vi "UI_Progress.vi"(8 "error in (no error)":errorcluster, 11 "Progress in":refnum<class "Progress.lvclass">) -> (0 "error out":errorcluster, 3 "Progress out":refnum<class "Progress.lvclass">)   [LabVIEW 2021, in "Progress.lvlib" / "Progress.lvclass"]
uses:
  Progress.lvclass
panel:
  out "Slide":u64(slide) scale=0.0..1.0
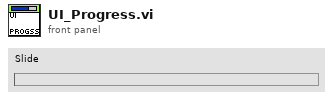
[diagram p1: front panel]
types:
  T1 = enum32{"Invalid", "Standard", "Closed", "Hidden", "Minimized", "Maximized"}
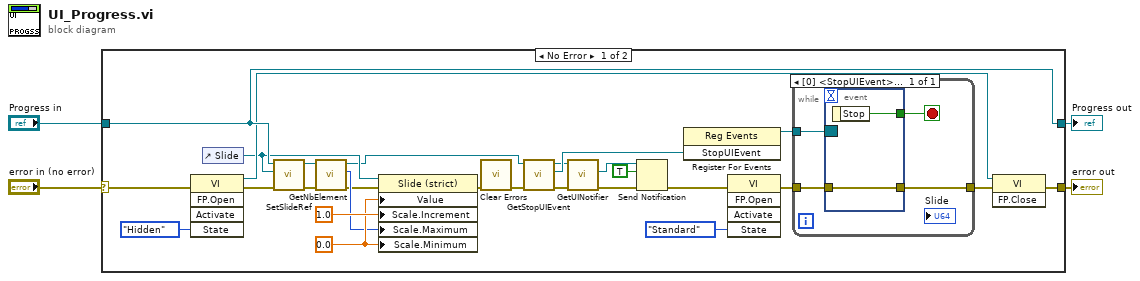
[diagram p0: block diagram]
diagram:
  n1 = case shown="No Error" "error in (no error)" {
    selector: "error in (no error)" -> [w16 w39]
    tunnel: [w15 w39] -> w3
    tunnel: [w31 w38] -> w1
    tunnel: "Progress in" -> [w31 w38]
    frame No Error {
      w13 = 0.0 ("ProgressValue")
      n2 = invoke class="VI" method="FP.Open"(error in=w16, "State"=T1."Hidden") -> (reference out=w18:refnum<vi>, error out=w19:errorcluster)  [unwired: 3 in, 3 out]
      n3 = control-ref of="Slide"() -> (w12:refnum<vi>)
      n4 = call "SetSlideRef.vi"("error in (no error)"=w19, "SlideRefnum"=w12, "Progress in"=w31) -> ("error out"=w11:errorcluster, "Progress out"=w10:refnum<class "Progress.lvclass">)  [unwired: 7 in]
      n5 = call "GetNbElement.vi"("error in (no error)"=w11, "Progress in"=w10) -> ("error out"=w6:errorcluster, "NbElement"=w9:u64, "Progress out"=w7:refnum<class "Progress.lvclass">)  [unwired: 7 in]
      n6 = property class="Slide (strict)"(reference=w12, error in=w6, "Value"=w13, "Scale.Increment"=1.0 ("Scale.Range:Increment"), "Scale.Maximum"=w9, "Scale.Minimum"=w13) -> (error out=w5:errorcluster)  [unwired: 1 out]
      n7 = call <vilib>:"Clear Errors.vi"("error in (no error)"=w5) -> ("error out"=w8:errorcluster)  [unwired: 5 in, 1 out]
      n8 = call "GetStopUIEvent.vi"("error in (no error)"=w8, "Progress in"=w7) -> ("error out"=w27:errorcluster, "StopUIEvent"=w28:refnum<user-event>, "Progress out"=w24:refnum<class "Progress.lvclass">)  [unwired: 7 in]
      n9 = call "GetUINotifier.vi"("error in (no error)"=w27, "Progress in"=w24) -> ("error out"=w26:errorcluster, "UINotifier"=w25:refnum<notifier>)  [unwired: 7 in, 1 out]
      n10 = Send Notification(notification=TRUE, notifier=w25, error in (no error)=w26) -> (error out=w21:errorcluster)  [unwired: 1 out]
      n11 = register-events(w28) -> (reference out=w29:refnum<event-registration>)  [unwired: 2 in, 1 out]
      n12 = invoke class="VI" method="FP.Open"(error in=w21, "State"=T1."Standard") -> (error out=w22:errorcluster)  [unwired: 3 in, 4 out]
      n13 = while {
        tunnel: w29 -> [w35]
        tunnel: w22 -> [w33]
        tunnel: [w32] -> w17
        stop <- w34 stop-if-true
        n14 = event shown="[0] <StopUIEvent>: User Event" {
          selector: w35 -> [_]
          dyn-events: _ -> [_]
          timeout: _ -> [_]
          tunnel: [w37] -> w34
          tunnel: w33 -> [w36]
          tunnel: [w36] -> w32
          event User Event {
            n15 = event-data() -> ("Stop"=w37:bool)  [unwired: 1 in]
          }
        }
      }
      n16 = invoke class="VI" method="FP.Close"(reference=w18, error in=w17) -> (error out=w15:errorcluster)  [unwired: 1 in, 2 out]
    }
    frame Error {
    }
  }
  "error out" <- w3
  "Progress out" <- w1
